vi "test-quintic-spline-01.vi"() -> ()   [LabVIEW 2019]
uses:
  <vilib>/Rock Robotics/WPI/ThirdParty/JAS_Junk/TrajLib/POSEwCURVATURE.ctl
  <vilib>/Rock Robotics/WPI/ThirdParty/JAS_Junk/TrajLib/POSE2D.ctl
  <vilib>/Rock Robotics/WPI/ThirdParty/JAS_Junk/TrajLib/TRANSLATION2D.ctl
  <vilib>/Rock Robotics/WPI/ThirdParty/JAS_Junk/TrajLib/ROTATION2D.ctl
  <vilib>/Rock Robotics/WPI/ThirdParty/JAS_Junk/TrajLib/Rotation_CreateAngle.vi
  <vilib>/Rock Robotics/WPI/ThirdParty/JAS_Junk/TrajLib/Translation_Create.vi
  <vilib>/Rock Robotics/WPI/ThirdParty/JAS_Junk/TrajLib/Util_CalcDist.vi
  <vilib>/Rock Robotics/WPI/ThirdParty/JAS_Junk/TrajLib/Trajectory_Library.lvlib
panel:
  out "XY Graph":cluster{dbl[], dbl[]}(graph)
  out "Numb\nWaypoints":i32
  out "All Interior \nwayPoints\nFound (True)":bool
  out "end rot = 0":dbl
  out "end y = 0":dbl
  out "end x = 0":dbl
  out "start rot = 0":dbl
  out "start y = 0":dbl
  out "start x = 0":dbl
  out "max dtheta < 0.0872":dbl
  out "max dy < 0.00127":dbl
  out "max dx  < 0.127":dbl
  out "Overall Error":errorcluster
  out "Elements":i32
  out "Create Spline Error":errorcluster
  out "SplinePoses\nWCurve":T1[](array[typedef]) {"POSE"."ROTATION"."SIN" format="%13.4f"; "POSE"."ROTATION"."COS" format="%13.4f"; "POSE"."ROTATION"."VALUE" format="%13.4f"; "POSE"."TRANSLATION"."Y" format="%14.3f"; "POSE"."TRANSLATION"."X" format="%14.3f"}
  out "Elapsed Time":dbl
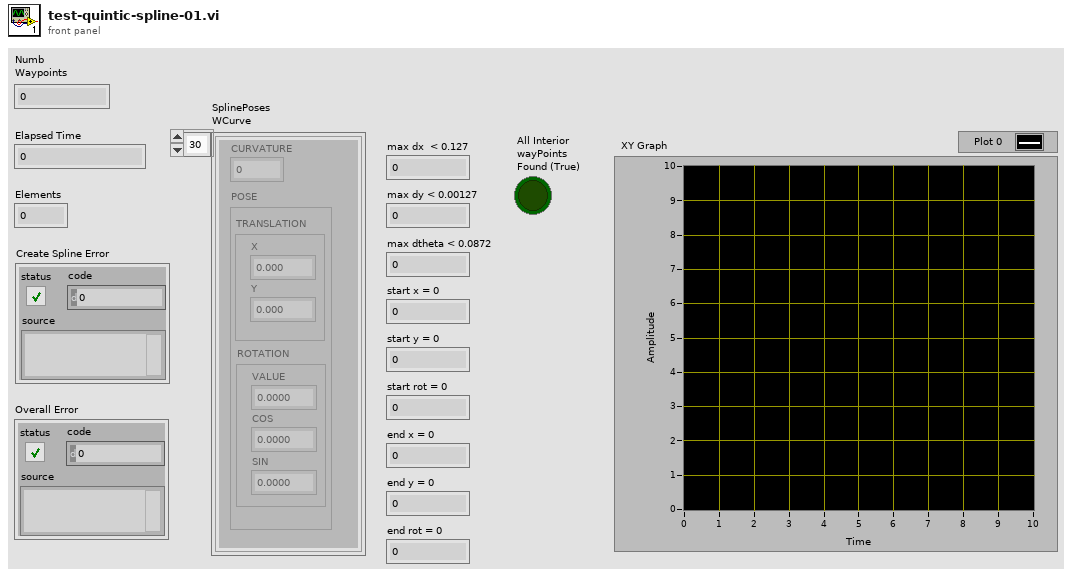
[diagram p1: front panel]
types:
  T1 = typedef "Trajectory_Library.lvlib/POSEwCURVATURE.ctl" = cluster{"CURVATURE":dbl, "POSE":T2}
  T2 = typedef "Trajectory_Library.lvlib/POSE2D.ctl" = cluster{"TRANSLATION":T3, "ROTATION":T4}
  T3 = typedef "Trajectory_Library.lvlib/TRANSLATION2D.ctl" = cluster{"X":dbl, "Y":dbl}
  T4 = typedef "Trajectory_Library.lvlib/ROTATION2D.ctl" = cluster{"VALUE":dbl, "COS":dbl, "SIN":dbl}
  T5 = typedef "Trajectory_Library.lvlib/SPLINE_CTRL_VECTOR.ctl" = cluster{"Xs":dbl[], "Ys":dbl[]}
  T6 = typedef "Trajectory_Library.lvlib/SPLINE.ctl" = cluster{"Degree":i32, "Coefficients":T7}
  T7 = typedef "NI_Matrix.lvlib/RealMatrix.ctl" = dbl[][]
  T8 = typedef "Trajectory_Library.lvlib/TWIST2D.ctl" = cluster{"dX":dbl, "dY":dbl, "dTHETA":dbl}
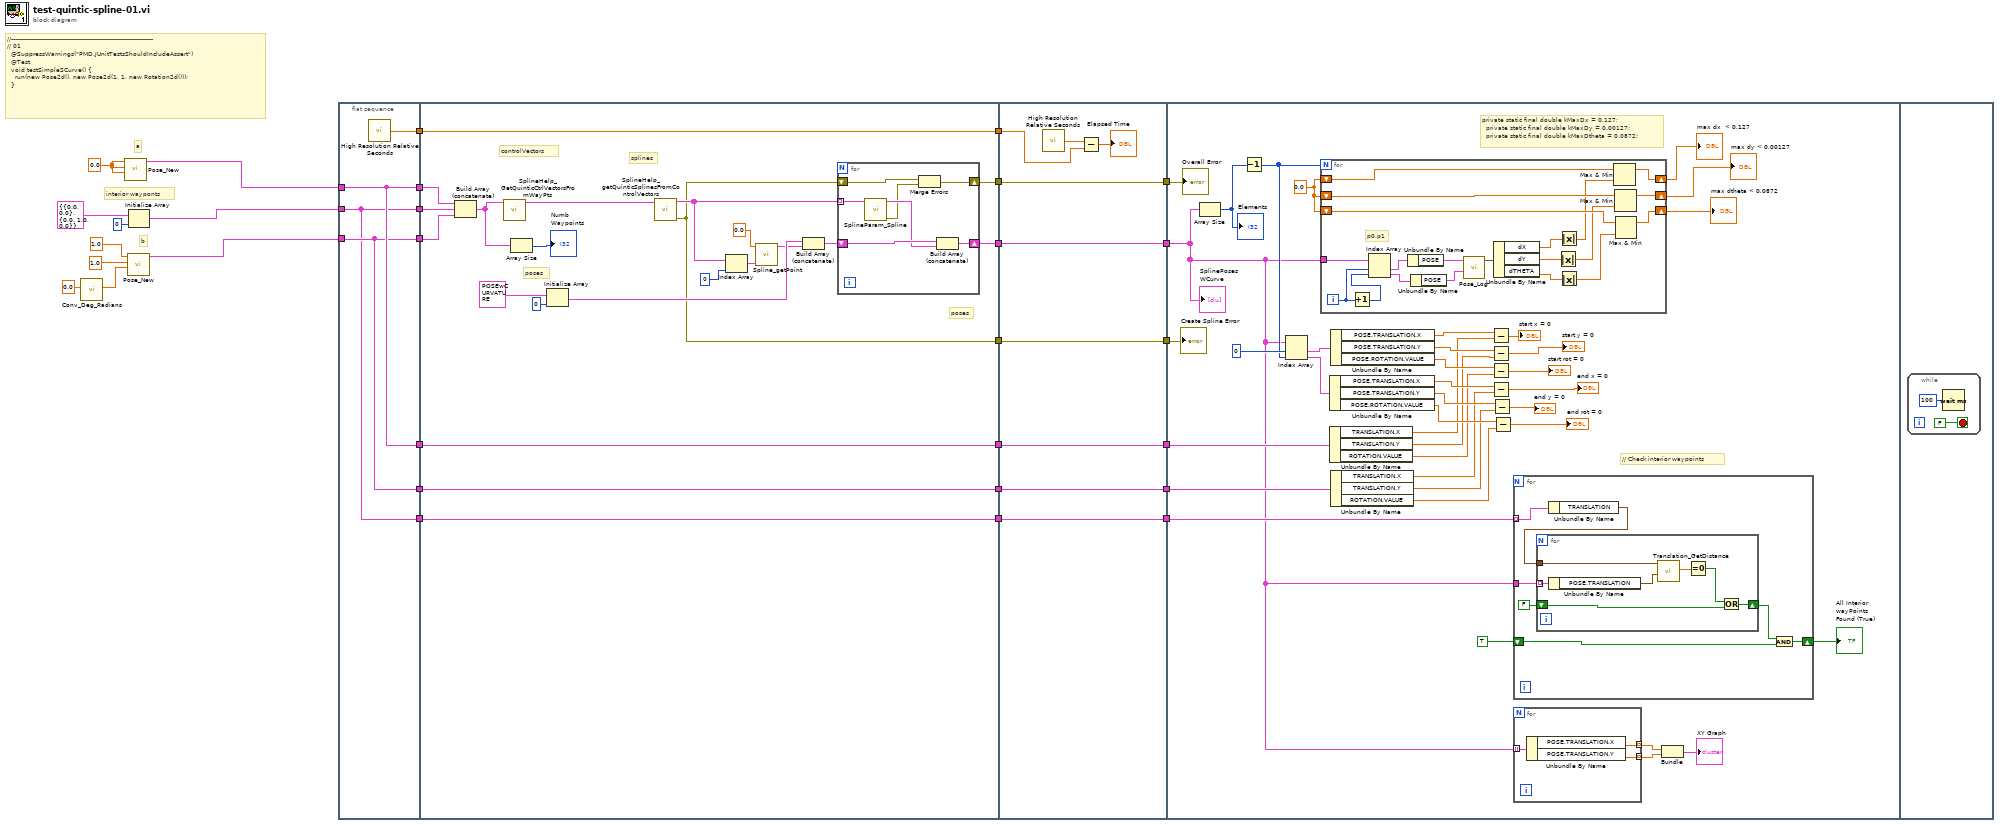
[diagram p0: block diagram]
diagram:
  w30 = 0.0 ("X")
  # "interior wayponts"
  # "b"
  # "a"
  # "//-----------------------------------------------------------------------\n// 01\n  @SuppressWarnings(\"PMD.JUnitTestsShouldIncludeAssert\")\n  @Test\n  void testSimpleSCurve() {\n    run(new Pose2d(), new Pose2d(1, 1, new Rotation2d()));\n  }"
  n1 = call <vilib>:"Conv_Deg_Radians.vi"("Degress"=0.0) -> ("Radians"=w2:dbl)  [unwired: 10 in]
  n2 = call <vilib>:"Pose_New.vi"("Heading"=w30, "Y"=w30, "X"=w30) -> ("out POSe"=w29:T2)  [unwired: 8 in]
  n3 = call <vilib>:"Pose_New.vi"("Heading"=w2, "Y"=1.0, "X"=1.0) -> ("out POSe"=w27:T2)  [unwired: 8 in]
  n4 = Initialize Array(T2 {"TRANSLATION"={"X"=0.0, "Y"=0.0}, "ROTATION"={"VALUE"=0.0, "COS"=1.0, "SIN"=0.0}} ("POSE"), 0 ("dimension size")) -> (w6:T2[])
  n5 = flat-sequence {
    tunnel: w29 -> [w33]
    tunnel: [w33] -> w28
    tunnel: w27 -> [w32]
    tunnel: [w32] -> w26
    tunnel: [w34] -> w25
    tunnel: [w33] -> w17
    tunnel: [w32] -> w14
    tunnel: [w31] -> w9
    tunnel: w6 -> [w31]
    tunnel: [w31] -> w5
    tunnel: w28 -> [w40]
    tunnel: w26 -> [w38]
    tunnel: [w56] -> w24
    tunnel: w25 -> [w56]
    tunnel: [w46] -> w23
    tunnel: [w45] -> w21
    tunnel: [w44] -> w19
    tunnel: w17 -> [w43]
    tunnel: [w43] -> w16
    tunnel: w14 -> [w42]
    tunnel: [w42] -> w13
    tunnel: [w41] -> w10
    tunnel: w9 -> [w41]
    tunnel: w5 -> [w37]
    tunnel: w24 -> [w72]
    tunnel: w23 -> [w71]
    tunnel: [w71] -> w22
    tunnel: w21 -> [w70]
    tunnel: [w70] -> w20
    tunnel: w19 -> [w69]
    tunnel: [w69] -> w18
    tunnel: w16 -> [w66]
    tunnel: [w66] -> w15
    tunnel: w13 -> [w65]
    tunnel: [w65] -> w12
    tunnel: [w64] -> w11
    tunnel: w10 -> [w64]
    tunnel: w22 -> [w74]
    tunnel: w20 -> [w110]
    tunnel: w18 -> [w109]
    tunnel: w15 -> [w103]
    tunnel: w12 -> [w102]
    tunnel: w11 -> [w79]
    frame #0 {
      n6 = call <vilib>:"High Resolution Relative Seconds.vi"() -> ("relative seconds"=w34:dbl)
    }
    frame #1 {
      # "poses"
      # "poses"
      # "splines"
      # "controlVectors"
      n7 = Build Array (concatenate)(w40, w37, w38) -> (w36:T2[])
      n8 = call <vilib>:"SplineHelp_GetQuinticCtrlVectorsFromWayPts.vi"("WayPoints"=w36) -> ("SplineControlVectors"=w39:T5[])  [unwired: 10 in]
      n9 = Array Size(array=w36) -> (size(s)=→"Numb\nWaypoints":i32)
      n10 = Initialize Array(T1 {"CURVATURE"=0.0, "POSE"={"TRANSLATION"={"X"=0.0, "Y"=0.0}, "ROTATION"={"VALUE"=0.0, "COS"=1.0, "SIN"=0.0}}} ("POSEwCURVATURE"), 0 ("dimension size")) -> (w50:T1[])
      n11 = call <vilib>:"SplineHelp_getQuinticSplinesFromControlVectors.vi"("ControlVectors"=w39) -> ("error out"=w45:errorcluster, "splines"=w47:T6[])  [unwired: 9 in]
      n12 = Index Array(array=w47, index=0) -> (element=w52:T6)
      n13 = call <vilib>:"Spline_getPoint.vi"("inputSPLINE"=w52, "Time"=0.0) -> ("POSEwCURVATURE"=w49:T1)  [unwired: 9 in]
      n14 = Build Array (concatenate)(w50, w49) -> (w48:T1[])
      n15 = for {
        shift-right: [w60] -> w46
        shift-left: w48 -> [w62]
        tunnel: w47 -> [w63] mode=indexing
        shift-right: [w58] -> w44
        shift-left: w45 -> [w59]
        n16 = call <vilib>:"SplineParam_Spline.vi"("inputSPLINE"=w63) -> ("error out"=w57:errorcluster, "outputPOSEwCURVATURE"=w61:T1[])  [unwired: 9 in]
        n17 = Merge Errors(w59, w57) -> (w58:errorcluster)
        n18 = Build Array (concatenate)(w62, w61) -> (w60:T1[])
      }
    }
    frame #2 {
      n19 = call <vilib>:"High Resolution Relative Seconds.vi"() -> ("relative seconds"=w67:dbl)
      n20 = Subtract(x=w67, y=w72) -> (x-y=→"Elapsed Time":dbl)
    }
    frame #3 {
      w107 = 0.0
      # "// Check interior waypoints"
      # "private static final double kMaxDx = 0.127;\n  private static final double kMaxDy = 0.00127;\n  private static final double kMaxDtheta = 0.0872;"
      n21 = Array Size(array=w74) -> (size(s)=w108:i32)
      "Elements" <- w108
      n22 = Decrement(x=w108) -> (x-1=w100:i32)
      n23 = Index Array(array=w74, index #1=0 ("index"), index #2=w100) -> (element #1=w99:T1, element #2=w98:T1)
      n24 = for {
        N: w100 -> [_]
        tunnel: w74 -> [w145]
        shift-right: [w136] -> w106
        shift-left: w107 -> [w133]
        shift-right: [w134] -> w104
        shift-left: w107 -> [w131]
        shift-right: [w135] -> w105
        shift-left: w107 -> [w132]
        i -> [w147]
        # "p0,p1"
        n25 = Increment(x=w147) -> (x+1=w146:i32)
        n26 = Index Array(array=w145, index #1=w147, index #2=w146) -> (element #1=w144:T1, element #2=w143:T1)
        n27 = Unbundle By Name(w144) -> ("POSE"=w142:T2)
        n28 = Unbundle By Name(w143) -> ("POSE"=w141:T2)
        n29 = call <vilib>:"Pose_Log.vi"("end POSE"=w141, "in POSE"=w142) -> ("out TWIST"=w140:T8)  [unwired: 9 in]
        n30 = Unbundle By Name(w140) -> ("dX"=w137:dbl, "dY"=w138:dbl, "dTHETA"=w139:dbl)
        n31 = Absolute Value(x=w138) -> (abs(x)=w129:dbl)
        n32 = Absolute Value(x=w137) -> (abs(x)=w130:dbl)
        n33 = Absolute Value(x=w139) -> (abs(x)=w128:dbl)
        n34 = Max & Min(x=w133, y=w130) -> (max(x,y)=w136:dbl)  [unwired: 1 out]
        n35 = Max & Min(x=w132, y=w129) -> (max(x,y)=w135:dbl)  [unwired: 1 out]
        n36 = Max & Min(x=w131, y=w128) -> (max(x,y)=w134:dbl)  [unwired: 1 out]
      }
      "max dx  < 0.127" <- w106
      "max dy < 0.00127" <- w105
      "max dtheta < 0.0872" <- w104
      n37 = Unbundle By Name(w98) -> ("POSE.TRANSLATION.X"=w94:dbl, "POSE.TRANSLATION.Y"=w93:dbl, "POSE.ROTATION.VALUE"=w92:dbl)
      n38 = Unbundle By Name(w103) -> ("TRANSLATION.X"=w91:dbl, "TRANSLATION.Y"=w90:dbl, "ROTATION.VALUE"=w89:dbl)
      n39 = Unbundle By Name(w99) -> ("POSE.TRANSLATION.X"=w97:dbl, "POSE.TRANSLATION.Y"=w96:dbl, "POSE.ROTATION.VALUE"=w95:dbl)
      n40 = Unbundle By Name(w102) -> ("TRANSLATION.X"=w88:dbl, "TRANSLATION.Y"=w87:dbl, "ROTATION.VALUE"=w86:dbl)
      n41 = Subtract(x=w97, y=w91) -> (x-y=→"start x = 0":dbl)
      n42 = Subtract(x=w96, y=w90) -> (x-y=→"start y = 0":dbl)
      n43 = Subtract(x=w95, y=w89) -> (x-y=→"start rot = 0":dbl)
      n44 = Subtract(x=w94, y=w88) -> (x-y=→"end x = 0":dbl)
      n45 = Subtract(x=w93, y=w87) -> (x-y=→"end y = 0":dbl)
      n46 = Subtract(x=w92, y=w86) -> (x-y=→"end rot = 0":dbl)
      n47 = for {
        tunnel: w79 -> [w115] mode=indexing
        tunnel: w74 -> [w120]
        shift-right: [w119] -> w77
        shift-left: TRUE -> [w118]
        n48 = Unbundle By Name(w115) -> ("TRANSLATION"=w114:T3)
        n49 = for {
          tunnel: w120 -> [w124] mode=indexing
          shift-right: [w127] -> w116
          shift-left: FALSE -> [w126]
          tunnel: w114 -> [w125]
          n50 = Unbundle By Name(w124) -> ("POSE.TRANSLATION"=w123:T3)
          n51 = call <vilib>:"Translation_GetDistance.vi"("other Translation"=w123, "In Translation"=w125) -> ("Distance"=w122:dbl)  [unwired: 9 in]
          n52 = Equal To 0?(x=w122) -> (x = 0?=w121:bool)
          n53 = Or(x=w121, y=w126) -> (x .or. y?=w127:bool)
        }
        n54 = And(x=w116, y=w118) -> (x .and. y?=w119:bool)
      }
      "All Interior \nwayPoints\nFound (True)" <- w77
      n55 = for {
        tunnel: [w113] -> w76 mode=indexing
        tunnel: [w112] -> w75 mode=indexing
        tunnel: w74 -> [w111] mode=indexing
        n56 = Unbundle By Name(w111) -> ("POSE.TRANSLATION.X"=w113:dbl, "POSE.TRANSLATION.Y"=w112:dbl)
      }
      n57 = Bundle(w76, w75) -> (→"XY Graph":cluster{dbl[], dbl[]})  [unwired: 1 in]
      "SplinePoses\nWCurve" <- w74
      "Create Spline Error" <- w110
      "Overall Error" <- w109
    }
    frame #4 {
      n58 = while {
        stop <- FALSE stop-if-true
        n59 = Wait (ms)(milliseconds to wait=u32 100) -> ()  [unwired: 1 out]
      }
    }
  }
